vi "Spectrograph_issueCommand_homeLinearStage.vi"(8 "error in (no error)":errorcluster, 11 "command_homeLinearStage_Ctl":T1) -> (0 "error out":errorcluster, 2 "function return":i32, 3 "command_homeLinearStage_Ctl out":T1)   [LabVIEW 2016, in "SALLV_Spectrograph.lvlib"]
doc: "int Spectrograph_shm_issueCommand_homeLinearStageLV(Spectrograph_command_homeLinearStageLV *command_homeLinearStage_Ctl );"
uses:
  SALLV_Spectrograph.lvlib
  DataTypes/command_homeLinearStage.ctl
  SALLV_Spectrograph.so
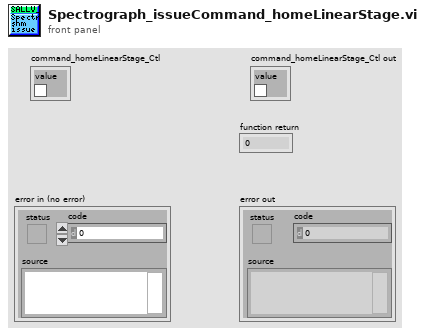
[diagram p1: front panel]
types:
  T1 = typedef "SALLV_Spectrograph.lvlib/command_homeLinearStage.ctl" = cluster{"value":bool}
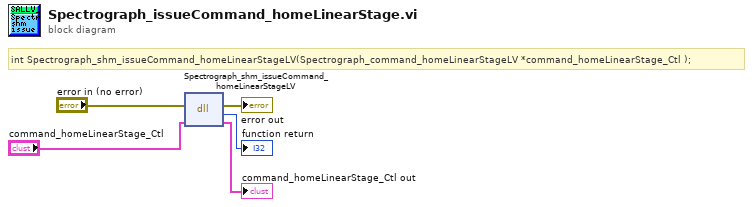
[diagram p0: block diagram]
diagram:
  # "int Spectrograph_shm_issueCommand_homeLinearStageLV(Spectrograph_command_homeLinearStageLV *command_homeLinearStage_Ctl );"
  n1 = dll-call lib="home/harini/TCS/SALLV_Spectrograph/SALLV_Spectrograph.*" fn="Spectrograph_shm_issueCommand_homeLinearStageLV"(error in="error in (no error)", "command_homeLinearStage_Ctl"="command_homeLinearStage_Ctl") -> (error out=→"error out":errorcluster, →"function return":i32, "command_homeLinearStage_Ctl"=→"command_homeLinearStage_Ctl out":T1)  [unwired: 2 in, 1 out]
